vi "InitAndEmptyImageBuffer.vi"(6 "FPGA.SEin":T1, 7 "Saving buffer":enum16{"main", "aux"}(ring)=enum."aux", 8 "error in (no error)":errorcluster, 9 "Requested Depth":u32, 10 "Timeout (ms)":i32=20, 11 "Refnum in":T2) -> (0 "error out":errorcluster, 3 "Refnum Out":T2, 4 "FPGA.SEout":T1)   [LabVIEW 2016]
uses:
  controls/FPGAVIreferenceTypeDef.ctl
  controls/FPGAVIreferenceTypeDefScanEngine.ctl
  <vilib>/Utility/error.llb/Error Cluster From Error Code.vi
  <vilib>/rvi/errors/niLvFpgaAdjustHostInterfaceError.vi
  <vilib>/rvi/interface/common/niFpgaWaitOnOcc.vi
  <vilib>/rvi/interface/nirviReadWriteControl/nirviReadWriteControl.xnode
  FPGA Bitfiles/qnmController797_usbRIO_controllerFPGAmu.lvbitx
  <vilib>/rvi/interface/nirviMethod/nirviMethod.xnode
  <vilib>/rvi/errors/niLvFpgaMergeErrorWithErrorCode.vi
  NiFpgaLv.dll
  <vilib>/FPGAPlugInAG/USB-7856R OEM/niLvFpga_ConfigureFifo_USB-7856R OEM.vi
  <vilib>/FPGAPlugInAG/USB-7856R OEM/niLvFpga_ReadFifo_USB-7856R OEM.vi
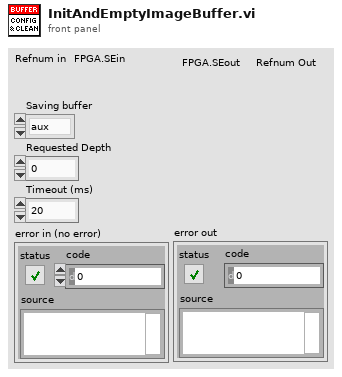
[diagram p1: front panel]
types:
  T1 = typedef "FPGAVIreferenceTypeDefScanEngine.ctl" = refnum<k20>
  T2 = typedef "FPGAVIreferenceTypeDef.ctl" = refnum<k20>
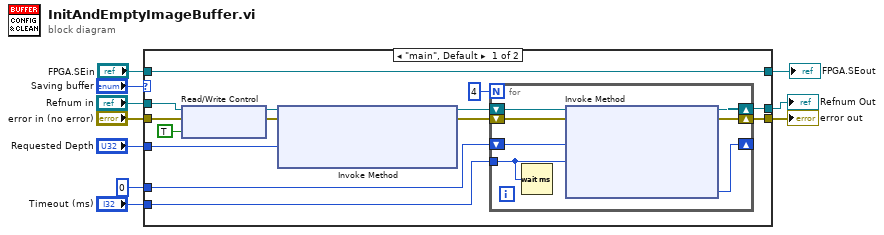
[diagram p0: block diagram]
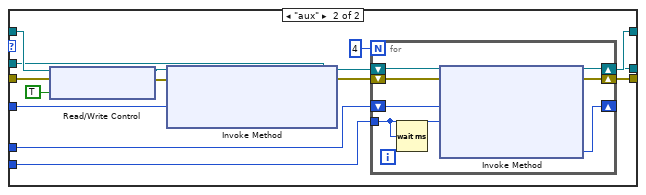
[diagram p2: hidden frame]
diagram:
  n1 = case shown="\"main\", Default" "Saving buffer" {
    tunnel: [w13 w37] -> w10
    tunnel: "Refnum in" -> [w16 w32]
    tunnel: "Timeout (ms)" -> [w20 w36]
    tunnel: u32 0 ("Number of Elements") -> [w19 w38]
    tunnel: "Requested Depth" -> [w18 w43]
    tunnel: "error in (no error)" -> [w17 w40]
    tunnel: [w14 w32] -> w4
    tunnel: "FPGA.SEin" -> [w11 w34]
    tunnel: [w11 w33] -> w1
    frame "main", Default {
      n2 = xnode "Read/Write Control"("FPGA VI Reference In"=w16, "error in"=w17, "hdt.o.enable"=TRUE) -> ("FPGA VI Reference Out"=w22:T2, "error out"=w21:errorcluster)
      n3 = xnode "Invoke Method"("FPGA VI Reference In"=w22, "error in"=w21, "Requested Depth"=w18) -> ("FPGA VI Reference Out"=w23:T2, "error out"=w24:errorcluster)  [unwired: 1 out]
      n4 = for {
        N: 4 -> [_]
        tunnel: w20 -> [w25]
        shift-right: [w28] -> w13
        shift-left: w24 -> [w31]
        shift-right: [w29] -> w14
        shift-left: w23 -> [w30]
        shift-right: [w27] -> _
        shift-left: w19 -> [w26]
        n5 = Wait (ms)(milliseconds to wait=w25) -> ()  [unwired: 1 out]
        n6 = xnode "Invoke Method"("FPGA VI Reference In"=w30, "error in"=w31, "Number of Elements"=w26, "Timeout (ms)"=w25) -> ("FPGA VI Reference Out"=w29:T2, "error out"=w28:errorcluster, "Elements Remaining"=w27:u32)  [unwired: 1 out]
      }
    }
    frame "aux" {
      n7 = xnode "Read/Write Control"("FPGA VI Reference In"=w34, "error in"=w40, "hdt.aux.o.enable"=TRUE) -> ("FPGA VI Reference Out"=w41:T1, "error out"=w42:errorcluster)
      n8 = xnode "Invoke Method"("FPGA VI Reference In"=w41, "error in"=w42, "Requested Depth"=w43) -> ("FPGA VI Reference Out"=w44:T1, "error out"=w45:errorcluster)  [unwired: 1 out]
      n9 = for {
        N: 4 -> [_]
        tunnel: w36 -> [w46]
        shift-right: [w49] -> w37
        shift-left: w45 -> [w52]
        shift-right: [w50] -> w33
        shift-left: w44 -> [w51]
        shift-right: [w48] -> _
        shift-left: w38 -> [w47]
        n10 = Wait (ms)(milliseconds to wait=w46) -> ()  [unwired: 1 out]
        n11 = xnode "Invoke Method"("FPGA VI Reference In"=w51, "error in"=w52, "Number of Elements"=w47, "Timeout (ms)"=w46) -> ("FPGA VI Reference Out"=w50:T1, "error out"=w49:errorcluster, "Elements Remaining"=w48:u32)  [unwired: 1 out]
      }
    }
  }
  "error out" <- w10
  "Refnum Out" <- w4
  "FPGA.SEout" <- w1
